vi "照明光控制-12_test.vi"() -> ()   [LabVIEW 2018]
uses:
  <vilib>/Instr/_visa.llb/VISA Configure Serial Port (Instr).vi
panel:
  in  "照明光":bool
  in  "stop":bool
  in  "stop bits (10: 1 bit)":u16(ring)=10 items=["1.0"=10, "1.5"=15, "2.0"=20]
  in  "parity (0:none)":enum16{"None", "Odd", "Even", "Mark", "Space"}(ring)
  in  "data bits (8)":u16=8 min=5 max=8 step=1
  in  "baud rate":u32=9600 caption="baud rate (115200)" min=9600 max=115200
  in  "VISA resource name":refnum<visa-resource-name>="COM7"
  # "通讯数据（16进制）：\nA0 01 00 A1\t开灯\t（不反馈）\nA0 01 01 A2\t关灯\t（不反馈）\nA0 01 02 A3\t开灯\t（反馈 A0 01 00 A1）\nA0 01 03 A4\t关灯\t（反馈 A0 01 01 A2）\nA0 01 04 A5\t取反\t（反馈当前状态）\nA0 01 05 A6\t查询状态\t（反馈当前状态）"
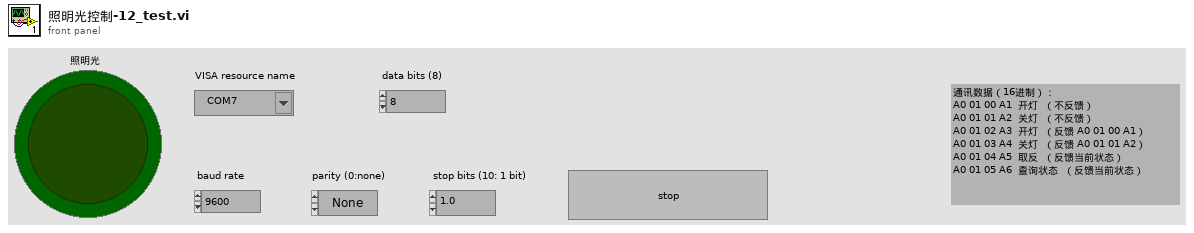
[diagram p1: front panel]
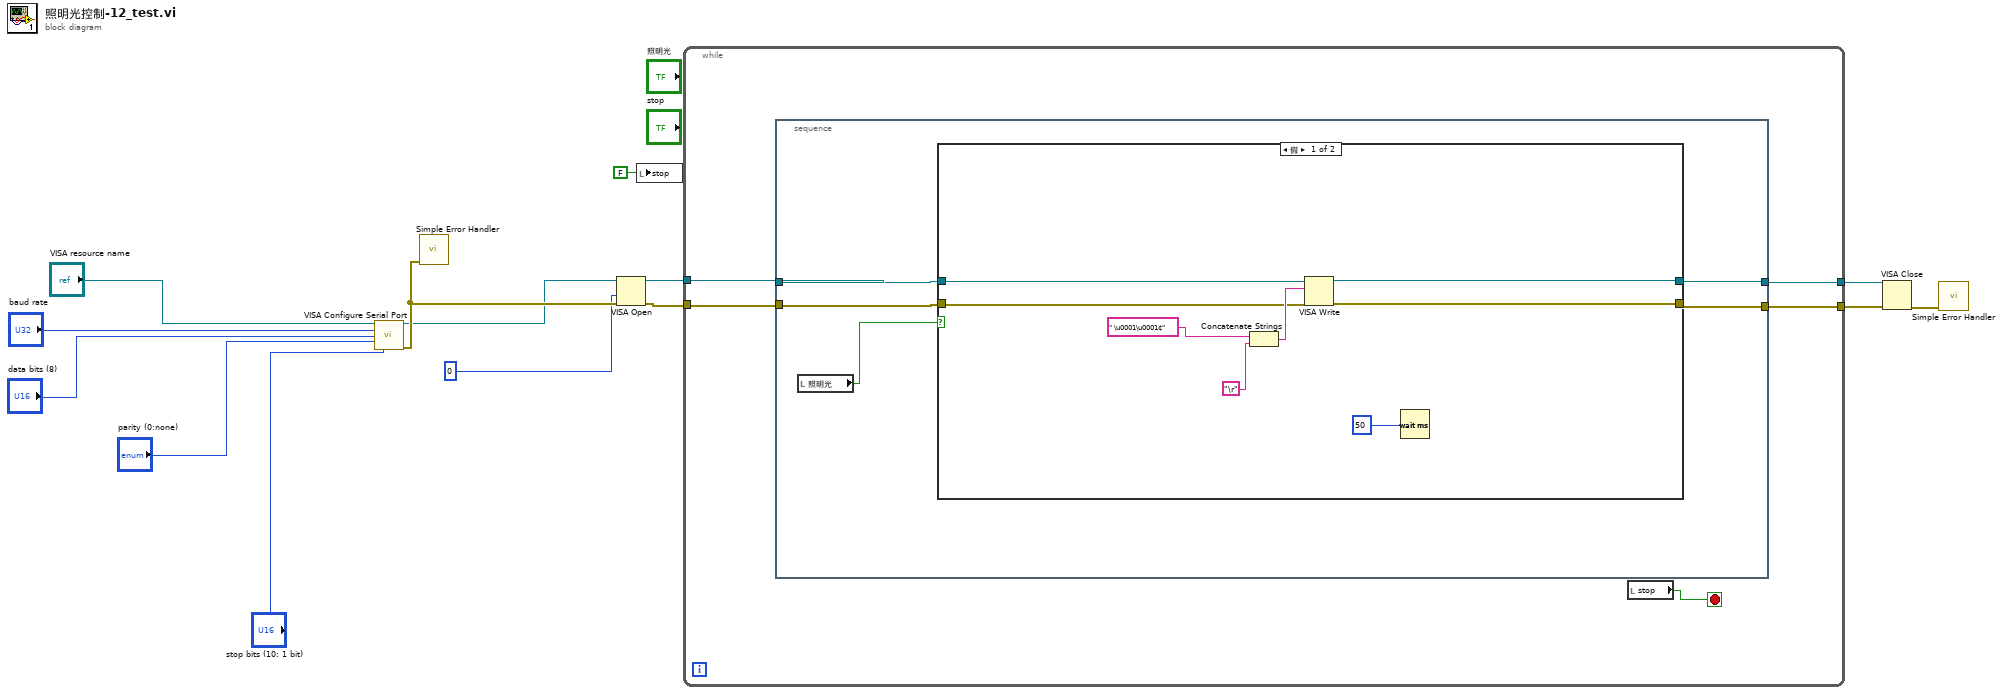
[diagram p0: block diagram]
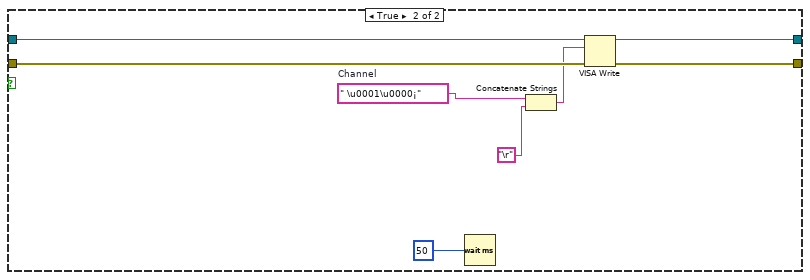
[diagram p2: hidden frame]
diagram:
  n1 = call-poly "VISA Configure Serial Port"("VISA resource name"="VISA resource name", "baud rate (9600)"="baud rate", "data bits (8)"="data bits (8)", "parity (0:none)"="parity (0:none)", "stop bits (10: 1 bit)"="stop bits (10: 1 bit)") -> ("VISA resource name out"=w3:refnum<visa-resource-name>, "error out"=w5:errorcluster)  [unwired: 9 in]
  n2 = call <vilib>:"Simple Error Handler.vi"("error in (no error)"=w5) -> ()  [unwired: 4 in, 5 out]
  n3 = VISA Open(access mode=0, error in (no error)=w5, VISA resource name=w3) -> (VISA resource name=w1:refnum<visa-resource-name>, error out=w2:errorcluster)  [unwired: 2 in]
  n4 = local write "stop"(FALSE ("stop")) -> ()
  n5 = while {
    tunnel: [w18] -> w7
    tunnel: [w17] -> w6
    tunnel: w2 -> [w16]
    tunnel: w1 -> [w15]
    stop <- w19 stop-if-true
    n6 = stacked-sequence {
      tunnel: w15 -> [w24]
      tunnel: w16 -> [w23]
      tunnel: [w21] -> w18
      tunnel: [w20] -> w17
      frame #0 {
        n7 = local read "照明光"() -> (w22:bool)
        n8 = case shown="假" w22 {
          tunnel: w24 -> [w30 w40]
          tunnel: [w28 w39] -> w21
          tunnel: w23 -> [w29 w38]
          tunnel: [w27 w37] -> w20
          frame False {
            n9 = Concatenate Strings(" \u0001\u0001¢", "\r") -> (w31:string)
            n10 = VISA Write(VISA resource name=w30, write buffer=w31, error in (no error)=w29) -> (VISA resource name out=w28:refnum<visa-resource-name>, error out=w27:errorcluster)  [unwired: 1 out]
            n11 = Wait (ms)(milliseconds to wait=50) -> ()  [unwired: 1 out]
          }
          frame True {
            w33 = " \u0001\u0000¡"  # Channel
            n12 = Wait (ms)(milliseconds to wait=50) -> ()  [unwired: 1 out]
            n13 = Concatenate Strings(w33, "\r") -> (w34:string)
            n14 = VISA Write(VISA resource name=w40, write buffer=w34, error in (no error)=w38) -> (VISA resource name out=w39:refnum<visa-resource-name>, error out=w37:errorcluster)  [unwired: 1 out]
          }
        }
      }
    }
    n15 = local read "stop"() -> (w19:bool)
  }
  n16 = VISA Close(VISA resource name=w7, error in (no error)=w6) -> (error out=w9:errorcluster)
  n17 = call <vilib>:"Simple Error Handler.vi"("error in (no error)"=w9) -> ()  [unwired: 4 in, 5 out]
